vi "ADAM_to_Eng_units.vi"(3 "Ch Description":T1={"Ch Name"="", "Type"="", "Function"=enum."Analogue Input", "Ch State"=enum."On", "Calibration type"="", "A"=0.0, "B"=0.0, "C"=0.0, "D"=0.0, "Comments"="", "Address"={"Main"=0, "Ch."=0, "Sub"=0, "Port Name"=""}, "String"="", "Duty"=65535} {"Duty" format="%016b"; "D" format="%#_5g"; "C" format="%#_5g"; "B" format="%#_5g"; "A" format="%#_5g"}, 5 "Raw":dbl format="%.2f") -> (1 "Calibrated units":dbl format="%.2f", 2 "Comments":string)   [LabVIEW 2016]
uses:
  ADAM Client/Sub VIs/ADAM Controls/Ch_description_ADAM.ctl
  ADAM Client/Sub VIs/ADAM Controls/Module_type_ADAM.ctl
  ADAM Client/Sub VIs/ADAM Controls/Function_ADAM.ctl
  ADAM Client/Sub VIs/ADAM Controls/Channel_State.ctl
  ADAM Client/Sub VIs/ADAM Controls/Calib_type_ADAM.ctl
  ADAM Client/Sub VIs/ADAM Controls/Address.ctl
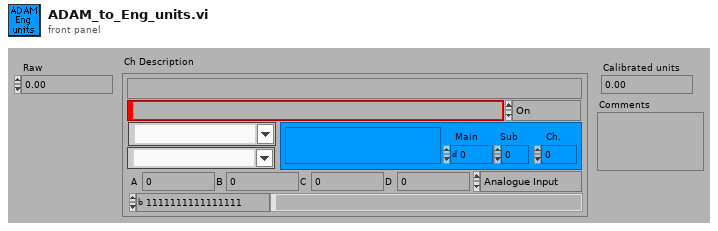
[diagram p1: front panel]
types:
  T1 = typedef "Ch_description_ADAM.ctl" = cluster{"Ch Name":string, "Type":T2, "Function":T3, "Ch State":T4, "Calibration type":T5, "A":dbl, "B":dbl, "C":dbl, "D":dbl, "Comments":string, "Address":T6, "String":string, "Duty":u16}
  T2 = typedef "Module_type_ADAM.ctl" = string
  T3 = typedef "Function_ADAM.ctl" = enum16{"Analogue Input", "Digital Input", "Event counter", "Event rate", "Analogue Output", "Digital Output", "Relay Output"}
  T4 = typedef "Channel_State.ctl" = enum16{"On", "Off", "Always On", "Always Off"}
  T5 = typedef "Calib_type_ADAM.ctl" = string
  T6 = typedef "Address.ctl" = cluster{"Main":i32, "Ch.":i32, "Sub":i32, "Port Name":string}
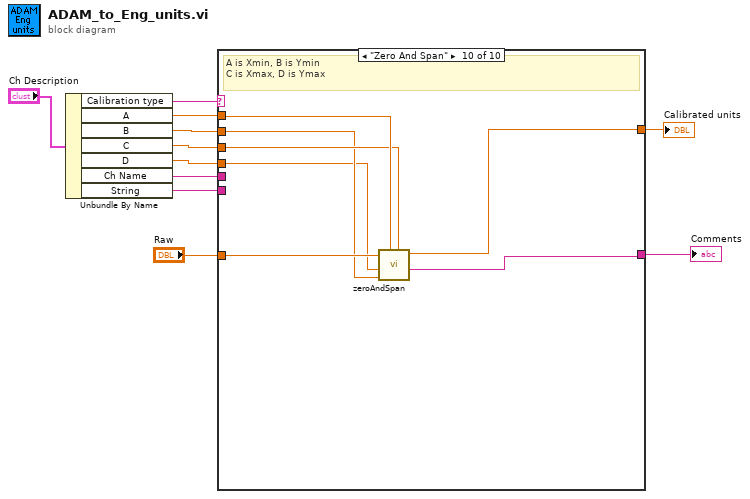
[diagram p0: block diagram]
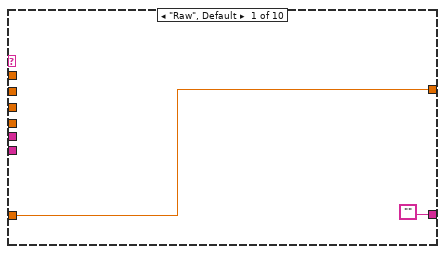
[diagram p2: hidden frame]
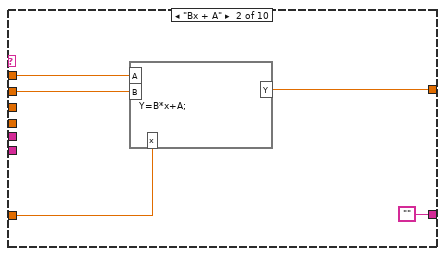
[diagram p3: hidden frame]
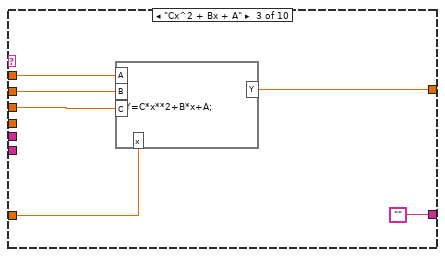
[diagram p4: hidden frame]
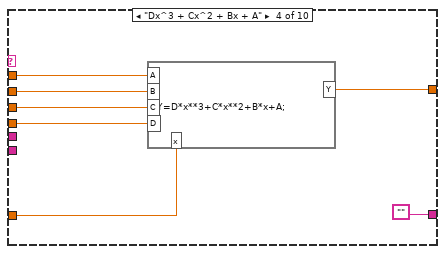
[diagram p5: hidden frame]
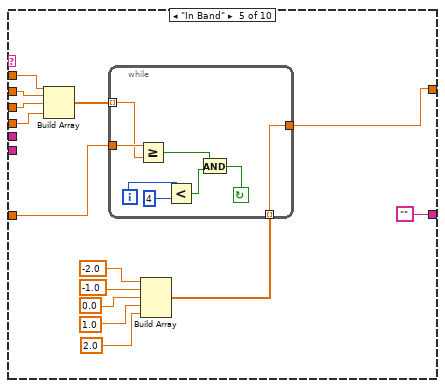
[diagram p6: hidden frame]
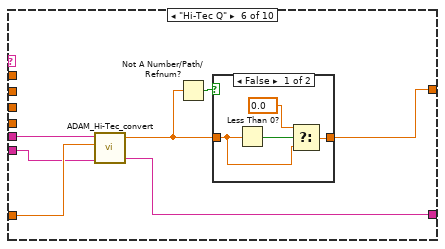
[diagram p7: hidden frame]
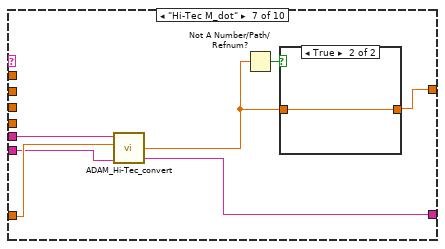
[diagram p9: hidden frame]
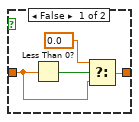
[diagram p10: hidden frame]
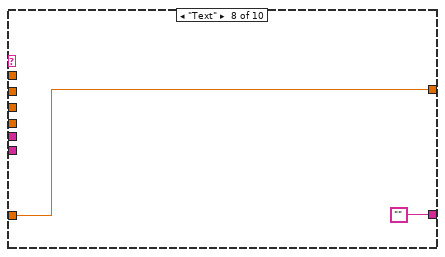
[diagram p11: hidden frame]
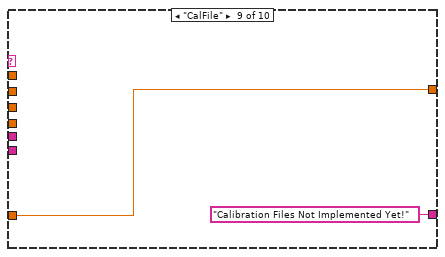
[diagram p12: hidden frame]
diagram:
  n1 = Unbundle By Name("Ch Description") -> ("Calibration type"=w10:T5, "A"=w7:dbl, "B"=w6:dbl, "C"=w5:dbl, "D"=w4:dbl, "Ch Name"=w3:string, "String"=w1:string)
  n2 = case shown="\"Zero And Span\"" w10 {
    tunnel: [w13 w18 w24 w31 w34 w57 w69 w79 w81 w86] -> w9
    tunnel: "Raw" -> [w13 w15 w20 w26 w41 w59 w71 w79 w81 w88]
    tunnel: w7 -> [_ w17 w23 w30 w45 _ _ _ _ w85]
    tunnel: w6 -> [_ w16 w22 w29 w44 _ _ _ _ w83]
    tunnel: w5 -> [_ _ w21 w28 w43 _ _ _ _ w84]
    tunnel: w4 -> [_ _ _ w27 w42 _ _ _ _ w82]
    tunnel: w3 -> [_ _ _ _ _ w60 w72 _ _ _]
    tunnel: ["" "" "" "" "" w55 w67 "" "Calibration Files Not Implemented Yet!" ("Comments") w87] -> w2
    tunnel: w1 -> [_ _ _ _ _ w54 w66 _ _ _]
    frame "Raw", Default {
    }
    frame "Bx + A" {
      n3 = formula code="Y=B*x+A;"("A"=w17, "B"=w16, "x"=w15) -> ("Y"=w18:dbl)
    }
    frame "Cx^2 + Bx + A" {
      n4 = formula code="Y=C*x**2+B*x+A;"("A"=w23, "B"=w22, "C"=w21, "x"=w20) -> ("Y"=w24:dbl)
    }
    frame "Dx^3 + Cx^2 + Bx + A" {
      n5 = formula code="Y=D*x**3+C*x**2+B*x+A;"("A"=w30, "B"=w29, "C"=w28, "D"=w27, "x"=w26) -> ("Y"=w31:dbl)
    }
    frame "In Band" {
      n6 = Build Array(w45, w44, w43, w42) -> (w40:dbl[])
      n7 = Build Array(-2.0, -1.0, 0.0, 1.0, 2.0) -> (w33:dbl[])
      n8 = while {
        tunnel: w33 -> [w51] mode=indexing
        tunnel: [w51] -> w34
        tunnel: w40 -> [w52] mode=indexing
        tunnel: w41 -> [w53]
        i -> [w50]
        stop <- w46 continue-if-true
        n9 = Greater Or Equal?(x=w53, y=w52) -> (x >= y?=w47:bool)
        n10 = Less?(x=w50, y=4) -> (x < y?=w48:bool)
        n11 = And(x=w47, y=w48) -> (x .and. y?=w46:bool)
      }
    }
    frame "Hi-Tec Q" {
      n12 = call "ADAM_Hi-Tec_convert.vi"("Ch Name"=w60, "Raw"=w59, "Channel Read"=w54) -> ("Q release (l/min)"=w56:dbl, "Comments"=w55:string)  [unwired: 1 in, 2 out]
      n13 = Not A Number/Path/Refnum?(number/path/refnum=w56) -> (NaN/Path/Refnum?=w58:bool)
      n14 = case shown="False" w58 {
        tunnel: [w62 w65] -> w57
        tunnel: w56 -> [w63 w65]
        frame False {
          n15 = Less Than 0?(x=w63) -> (x < 0?=w64:bool)
          n16 = Select(t=0.0, s=w64, f=w63) -> (s? t:f=w62:dbl)
        }
        frame True {
        }
      }
    }
    frame "Hi-Tec M_dot" {
      n17 = call "ADAM_Hi-Tec_convert.vi"("Ch Name"=w72, "Raw"=w71, "Channel Read"=w66) -> ("M_dot (kg/min)"=w68:dbl, "Comments"=w67:string)  [unwired: 1 in, 2 out]
      n18 = Not A Number/Path/Refnum?(number/path/refnum=w68) -> (NaN/Path/Refnum?=w70:bool)
      n19 = case shown="True" w70 {
        tunnel: [w74 w77] -> w69
        tunnel: w68 -> [w75 w77]
        frame False {
          n20 = Less Than 0?(x=w75) -> (x < 0?=w76:bool)
          n21 = Select(t=0.0, s=w76, f=w75) -> (s? t:f=w74:dbl)
        }
        frame True {
        }
      }
    }
    frame "Text" {
    }
    frame "CalFile" {
    }
    frame "Zero And Span" {
      # "A is Xmin, B is Ymin\nC is Xmax, D is Ymax"
      n22 = call "zeroAndSpan.vi"("Xmax"=w84, "Xmin"=w85, "Ymin"=w83, "Ymax"=w82, "MeasuredX"=w88) -> ("Message"=w87:string, "calibratedY"=w86:dbl)  [unwired: 4 in, 1 out]
    }
  }
  "Calibrated units" <- w9
  "Comments" <- w2
